vi "SendUserEvent.vi"(9 "error in (no error)":errorcluster, 10 "Message Cluster":T2, 11 "User Event in":refnum<user-event>) -> (1 "error out":errorcluster)   [LabVIEW 2018]
doc: "Permette l'invio degli user event in broadcast."
uses:
  Desktop/StateMachineTest/2/Messages.ctl
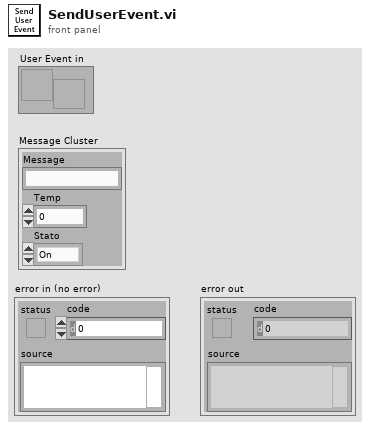
[diagram p1: front panel]
types:
  T1 = typedef "Messages.ctl" = string
  T2 = cluster{"Message":T1, "Temp":i32, "Stato":enum16{"On", "Off", "Preparation", "WaitTimer", "Ready"}}
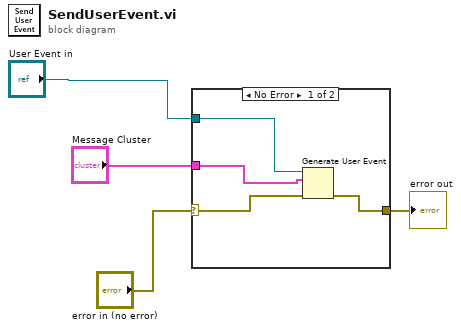
[diagram p0: block diagram]
diagram:
  n1 = case shown="No Error" "error in (no error)" {
    selector: "error in (no error)" -> [w7 w9]
    tunnel: [w8 w9] -> w3
    tunnel: "User Event in" -> [w6 _]
    tunnel: "Message Cluster" -> [w5 _]
    frame No Error {
      n2 = Generate User Event(user event=w6, event data cluster=w5, error in=w7) -> (error out=w8:errorcluster)  [unwired: 1 in, 1 out]
    }
    frame Error {
    }
  }
  "error out" <- w3
